vi "LowerRevisionHistoryCount.vi"() -> ()   [LabVIEW 2014]
panel:
  in  "History:Revision Number":u32
  in  "vi path":path
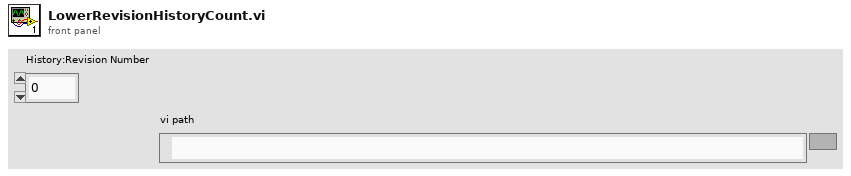
[diagram p1: front panel]
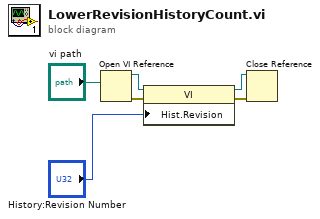
[diagram p0: block diagram]
diagram:
  n1 = Open VI Reference(vi path="vi path") -> (vi reference=w3:refnum<vi>, error out=w2:errorcluster)  [unwired: 5 in]
  n2 = property class="VI"(reference=w3, error in=w2, "Hist.Revision"="History:Revision Number") -> (reference out=w5:refnum<vi>, error out=w4:errorcluster)
  n3 = Close Reference(reference=w5, error in (no error)=w4) -> ()  [unwired: 1 out]
